vi "ValorAuto.vi"(11 "Steps":dbl[][](array[numeric])) -> ()   [LabVIEW 2017]
uses:
  Lift States.ctl
  Robot Global Data.vi
panel:
  in  "Max Drive Speed":dbl=0.2
  in  "Minimum Drive Speed":dbl=0.15
  out "Step Start Time":u32
  in  "First Time?":bool=TRUE
  in  "Step":i32
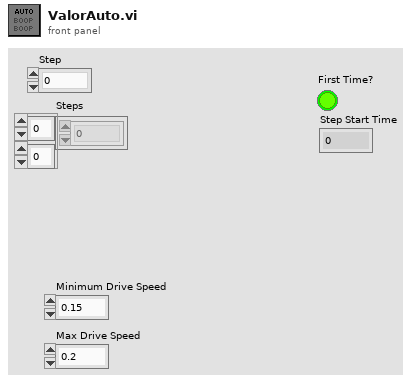
[diagram p1: front panel]
types:
  T1 = typedef "Auto Actions.ctl" = enum16{"Idle", "Drive", "Turn", "Lift", "Cube"}
  T2 = typedef "Lift States.ctl" = enum16{"Idle", "Hold Position", "Scale Low", "Scale Middle", "Scale High"}
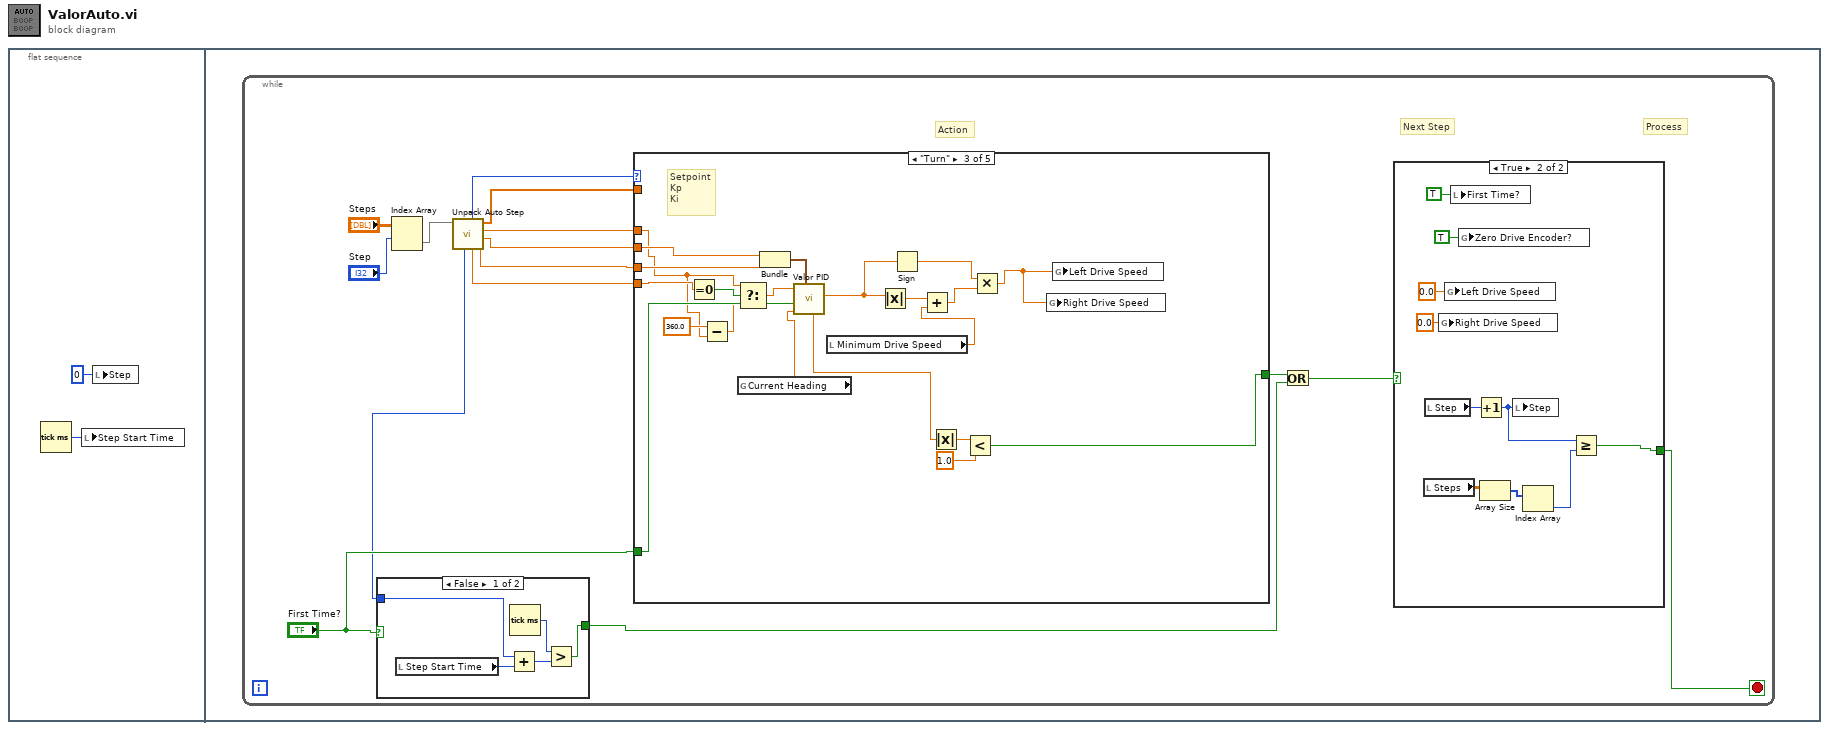
[diagram p0: block diagram]
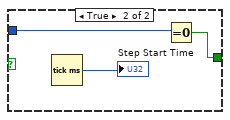
[diagram p2: hidden frame]
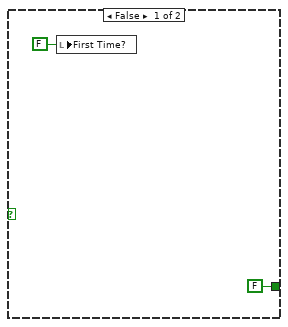
[diagram p3: hidden frame]
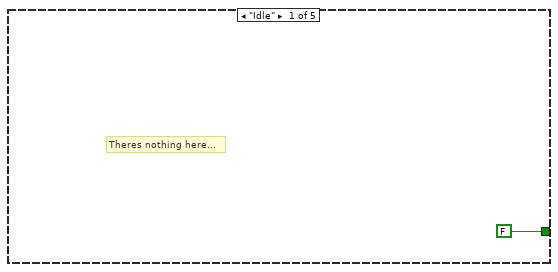
[diagram p4: hidden frame]
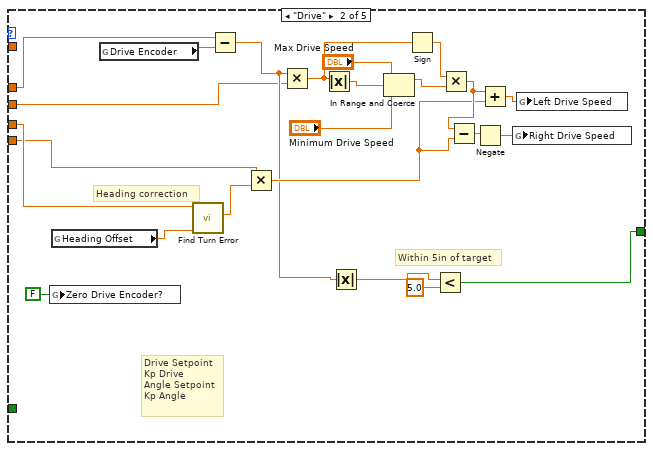
[diagram p5: hidden frame]
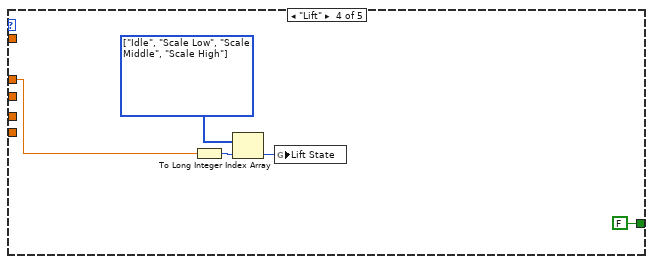
[diagram p6: hidden frame]
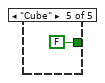
[diagram p7: hidden frame]
diagram:
  n1 = flat-sequence {
    frame #0 {
      n2 = Tick Count (ms)() -> (millisecond timer value=w1:u32)
      n3 = local write "Step Start Time"(w1) -> ()
      n4 = local write "Step"(0 ("Step")) -> ()
    }
    frame #1 {
      n5 = while {
        stop <- w12 stop-if-true
        # "Process"
        # "Next Step"
        # "Action"
        n6 = Index Array(array="Steps", index (row)="Step") -> (element=w10:dbl[])  [unwired: 1 in]
        n7 = call "Unpack Auto Step.vi"("Step Array"=w10) -> ("Arg3"=w6:dbl, "Arg2"=w7:dbl, "Arg1"=w8:dbl, "Args"=w9:dbl[], "Arg4"=w4:dbl, "Step Type"=w3:T1, "Timeout"=w5:u32)  [unwired: 4 in]
        n8 = case shown="False" "First Time?" {
          tunnel: [w19 w24] -> w14
          tunnel: w5 -> [w18 w23]
          frame False {
            n9 = local read "Step Start Time"() -> (w22:u32)
            n10 = Add(x=w18, y=w22) -> (x+y=w21:u32)
            n11 = Tick Count (ms)() -> (millisecond timer value=w20:u32)
            n12 = Greater?(x=w20, y=w21) -> (0:w19:bool)
          }
          frame True {
            n13 = Tick Count (ms)() -> (millisecond timer value=→"Step Start Time":u32)
            n14 = Equal To 0?(x=w23) -> (x = 0?=w24:bool)
          }
        }
        n15 = case shown="\"Turn\"" w3 {
          tunnel: [FALSE w47 w72 FALSE FALSE] -> w15
          tunnel: "First Time?" -> [_ _ w82 _ _]
          tunnel: w9 -> [_ _ _ _ _]
          tunnel: w8 -> [_ w42 w63 w84 _]
          tunnel: w7 -> [_ w41 w80 _ _]
          tunnel: w6 -> [_ w44 w79 _ _]
          tunnel: w4 -> [_ w43 w67 _ _]
          frame "Idle" {
            # "Theres nothing here..."
          }
          frame "Drive" {
            # "Drive Setpoint\nKp Drive\nAngle Setpoint\nKp Angle"
            # "Heading correction"
            # "Within 5in of target"
            n16 = global write "Robot Global Data.vi" "Zero Drive Encoder?"(FALSE ("Zero Drive Encoder?")) -> ()
            n17 = global read "Robot Global Data.vi" "Heading Offset"() -> (w60:dbl)
            n18 = global read "Robot Global Data.vi" "Drive Encoder"() -> (w61:dbl)
            n19 = call "Find Turn Error.vi"("Target Angle"=w44, "Current Angle"=w60) -> ("Error"=w59:dbl)  [unwired: 7 in]
            n20 = Subtract(x=w42, y=w61) -> (x-y=w46:dbl)
            n21 = Multiply(x=w43, y=w59) -> (x*y=w49:dbl)
            n22 = Multiply(x=w46, y=w41) -> (x*y=w55:dbl)
            n23 = Absolute Value(x=w55) -> (abs(x)=w56:dbl)
            n24 = Absolute Value(x=w46) -> (abs(x)=w45:dbl)
            n25 = In Range and Coerce(upper limit="Max Drive Speed", x=w56, lower limit="Minimum Drive Speed") -> (coerced(x)=w54:dbl)  [unwired: 1 out]
            n26 = Sign(1:w55) -> (0:w53:dbl)
            n27 = Less?(x=w45, y=5.0) -> (x < y?=w47:bool)
            n28 = Multiply(x=w53, y=w54) -> (x*y=w50:dbl)
            n29 = Subtract(x=w50, y=w49) -> (x-y=w51:dbl)
            n30 = Negate(x=w51) -> (-x=w58:dbl)
            n31 = Add(x=w50, y=w49) -> (x+y=w52:dbl)
            n32 = global write "Robot Global Data.vi" "Right Drive Speed"(w58) -> ()
            n33 = global write "Robot Global Data.vi" "Left Drive Speed"(w52) -> ()
          }
          frame "Turn" {
            # "Setpoint\nKp\nKi"
            n34 = Equal To 0?(x=w67) -> (x = 0?=w65:bool)
            n35 = Subtract(x=360.0, y=w63) -> (x-y=w62:dbl)
            n36 = Select(t=w63, s=w65, f=w62) -> (s? t:f=w66:dbl)
            n37 = global read "Robot Global Data.vi" "Current Heading"() -> (w81:dbl)
            n38 = Bundle("Arg2"=w80, "Arg3"=w79) -> (w78:cluster{"Arg2":dbl, "Arg3":dbl})  [unwired: 1 in]
            n39 = call "Valor PID.vi"("PI"=w78, "Current"=w81, "First Run"=w82, "Target"=w66) -> ("Output"=w71:dbl, "Error"=w75:dbl)  [unwired: 6 in]
            n40 = local read "Minimum Drive Speed"() -> (w69:dbl)
            n41 = Absolute Value(x=w71) -> (abs(x)=w70:dbl)
            n42 = Sign(1:w71) -> (0:w77:dbl)
            n43 = Add(x=w70, y=w69) -> (x+y=w68:dbl)
            n44 = Absolute Value(x=w75) -> (abs(x)=w74:dbl)
            n45 = Less?(x=w74, y=1.0) -> (x < y?=w72:bool)
            n46 = Multiply(x=w77, y=w68) -> (x*y=w76:dbl)
            n47 = global write "Robot Global Data.vi" "Right Drive Speed"(w76) -> ()
            n48 = global write "Robot Global Data.vi" "Left Drive Speed"(w76) -> ()
          }
          frame "Lift" {
            w86 = T2[] [enum."Idle", enum."Scale Low", enum."Scale Middle", enum."Scale High"] items=["Idle", "Hold Position", "Scale Low", "Scale Middle", "Scale High"]
            n49 = To Long Integer(number=w84) -> (32bit integer=w83:i32)
            n50 = Index Array(array=w86, index=w83) -> (element=w85:T2)
            n51 = global write "Robot Global Data.vi" "Lift State"(w85) -> ()
          }
          frame "Cube" {
          }
        }
        n52 = Or(x=w15, y=w14) -> (x .or. y?=w11:bool)
        n53 = case shown="True" w11 {
          tunnel: [FALSE w30] -> w12
          frame False {
            n54 = local write "First Time?"(FALSE ("First Time?")) -> ()
          }
          frame True {
            n55 = local read "Steps"() -> (w34:dbl[][])
            n56 = local read "Step"() -> (w35:i32)
            n57 = global write "Robot Global Data.vi" "Right Drive Speed"(0.0 ("Left Drive Speed")) -> ()
            n58 = global write "Robot Global Data.vi" "Left Drive Speed"(0.0 ("Left Drive Speed")) -> ()
            n59 = local write "First Time?"(TRUE ("First Time?")) -> ()
            n60 = global write "Robot Global Data.vi" "Zero Drive Encoder?"(TRUE ("Zero Drive Encoder?")) -> ()
            n61 = Increment(x=w35) -> (x+1=w29:i32)
            n62 = Array Size(array=w34) -> (size(s)=w33:i32[])
            n63 = local write "Step"(w29) -> ()
            n64 = Index Array(array=w33) -> (element=w28:i32)  [unwired: 1 in]
            n65 = Greater Or Equal?(x=w29, y=w28) -> (x >= y?=w30:bool)
          }
        }
      }
    }
  }
